vi "Tab Symbols.vi"(7 "Action (Get)":enum8{"Get", "Set"}(ring), 8 "error in (no error)":errorcluster, 10 "Symbol Image in":T1, 11 "Symbol Idx":i32) -> (0 "error out":errorcluster, 2 "Symbol Image out":T1, 3 "Indexes":i32[](array[numeric]))   [LabVIEW 2018, in "Tab.lvlib"]
uses:
  Tab.lvlib
  <vilib>/picture/picture.llb/imagedata.ctl
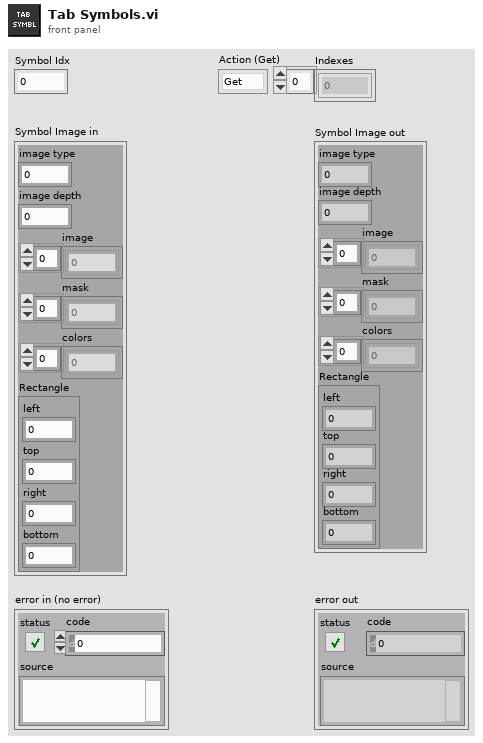
[diagram p1: front panel]
types:
  T1 = typedef "imagedata.ctl" = cluster{"image type":i32, "image depth":i32, "image":u8[], "mask":u8[], "colors":u32[], "Rectangle":cluster{"left":i16, "top":i16, "right":i16, "bottom":i16}}
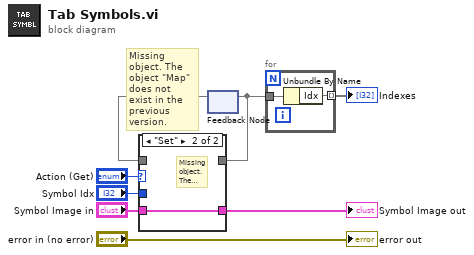
[diagram p0: block diagram]
diagram:
  # "Missing object. The object \"Map\" does not exist in the previous version."
  n1 = feedback #1() -> (w7, w3)
  n2 = case shown="\"Set\"" "Action (Get)" {
    tunnel: "Symbol Idx" -> [_ _]
    tunnel: [_ w11] -> w8
    tunnel: w7 -> [w10 w12]
    tunnel: [w10 _] -> w2
    tunnel: "Symbol Image in" -> [_ w11]
    frame "Get" {
      # "Missing object. The object \"Look In Map\" does not exist in the previous version."
    }
    frame "Set" {
      # "Missing object. The object \"Insert Into Map\" does not exist in the previous version."
    }
  }
  "Symbol Image out" <- w8
  n3 = feedback-in #1(w2) -> ()
  n4 = for {
    tunnel: w2 -> [w14]
    tunnel: [w13] -> w1 mode=indexing
    n5 = Unbundle By Name(w14) -> ("Idx"=w13)
  }
  "Indexes" <- w1
  "error out" <- "error in (no error)"
